vi "STAT2 decode Digital data from Solenoid node.vi"(10 "Solenoid Node Data":T2 {"valve status" format="%02x"; "sys register" format="%04x"}) -> (2 "Digital Data Out":T1[](array[typedef]))   [LabVIEW 2011]
uses:
  LEINmaster/Nodes/solonoid stat2.ctl
  Measurments Handling/Status Digitalish.ctl
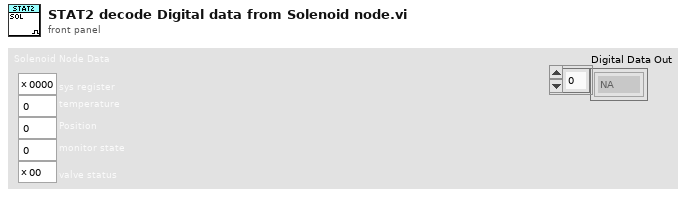
[diagram p1: front panel]
types:
  T1 = typedef "Status Digitalish.ctl" = enum16{"NA", "False", "True"}
  T2 = typedef "solonoid stat2.ctl" = cluster{"sys register":u16, "temperature":u16, "Position":i16, "monitor state":u8, "valve status":u8}
  T3 = typedef "Stat2 system error.ctl" = cluster{"Error":bool, "Has had error":bool, "Com. issue":bool}
  T4 = typedef "Stat2 system task info.ctl" = cluster{"Task":bool, "Task error":bool, "Task cnt.":u8, "Job 0":bool, "User":bool}
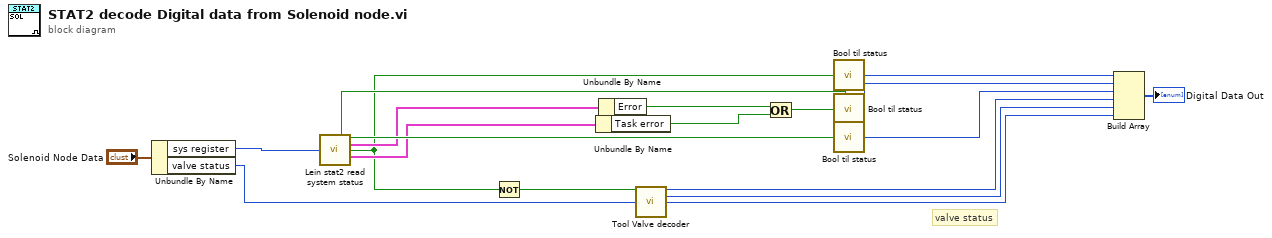
[diagram p0: block diagram]
diagram:
  # "valve status"
  n1 = Unbundle By Name("Solenoid Node Data") -> ("sys register"=w19:u16, "valve status"=w9:u8)
  n2 = call "Lein stat2 read system status.vi"("sys register"=w19) -> ("Force NA"=w12:bool, "Stopped"=w18:bool, "Error"=w14:T3, "Connected"=w8:bool, "Task"=w13:T4)  [unwired: 7 in, 3 out]
  n3 = Not(x=w8) -> (.not. x?=w7:bool)
  n4 = Unbundle By Name(w13) -> ("Task error"=w17:bool)
  n5 = Unbundle By Name(w14) -> ("Error"=w15:bool)
  n6 = call "Tool Valve decoder.vi"("Force NA(F)"=w7, "Valve Relay code"=w9) -> ("Valve LSB(0)"=w6:T1, "Valve 1"=w5:T1, "Valve 2"=w4:T1)  [unwired: 9 in, 2 out]
  n7 = Or(x=w15, y=w17) -> (x .or. y?=w16:bool)
  n8 = call "Bool til status.vi"("Boolean"=w8) -> ("Status"=w11:T1)  [unwired: 8 in]
  n9 = call "Bool til status.vi"("Force NA(F)"=w12, "Boolean"=w16) -> ("Status"=w2:T1)  [unwired: 7 in]
  n10 = call "Bool til status.vi"("Force NA(F)"=w12, "Boolean"=w18) -> ("Status"=w3:T1)  [unwired: 7 in]
  n11 = Build Array(w11, w2, w3, w6, w5, w4) -> (→"Digital Data Out":T1[])
